vi "Color Sensor V3 CIE sRGB Fcn.vi"(11 "Real Matrix Element":dbl) -> (3 "y":dbl)   [LabVIEW 2023]
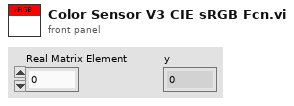
[diagram p1: front panel]
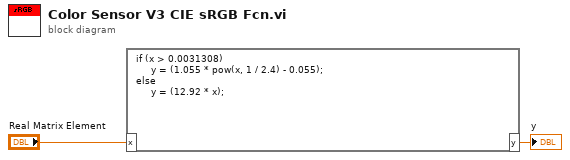
[diagram p0: block diagram]
diagram:
  n1 = formula code="if (x > 0.0031308)\n     y = (1.055 * pow(x, 1 / 2.4) - 0.055);\nelse\n     y = (12.92 * x);"("x"="Real Matrix Element") -> ("y"=→"y":dbl)
